vi "Tracker_v2_test_acq_comms_enq.vi"() -> ()   [LabVIEW 2018]
uses:
  Tracker.lvlib
panel:
  out "Data frame":T1
  out "Dequeued data frame":cluster{"String":string, timestamp}
  in  "Play/Pause":bool
  in  "Stop Button":bool
  out "Read buffer":string
  in  "VISA resource name in":refnum<visa-resource-name>="ASRL3::INSTR"
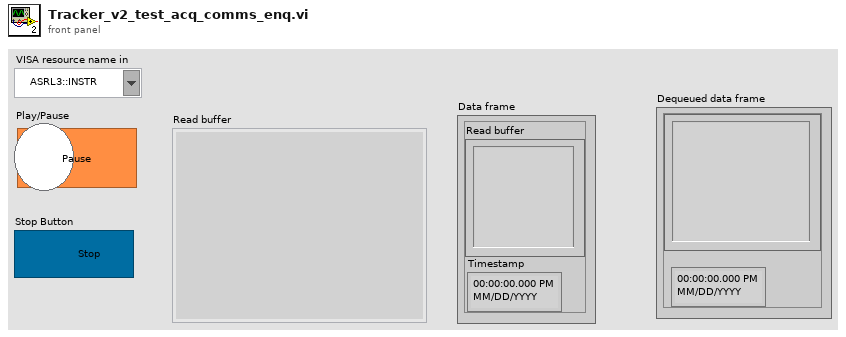
[diagram p1: front panel]
types:
  T1 = cluster{"Read buffer":string, "Timestamp":timestamp}
  T2 = cluster{"Data acquisition status":refnum<notifier>, "Play/Pause status":refnum<notifier>, "Recording status":refnum<notifier>}
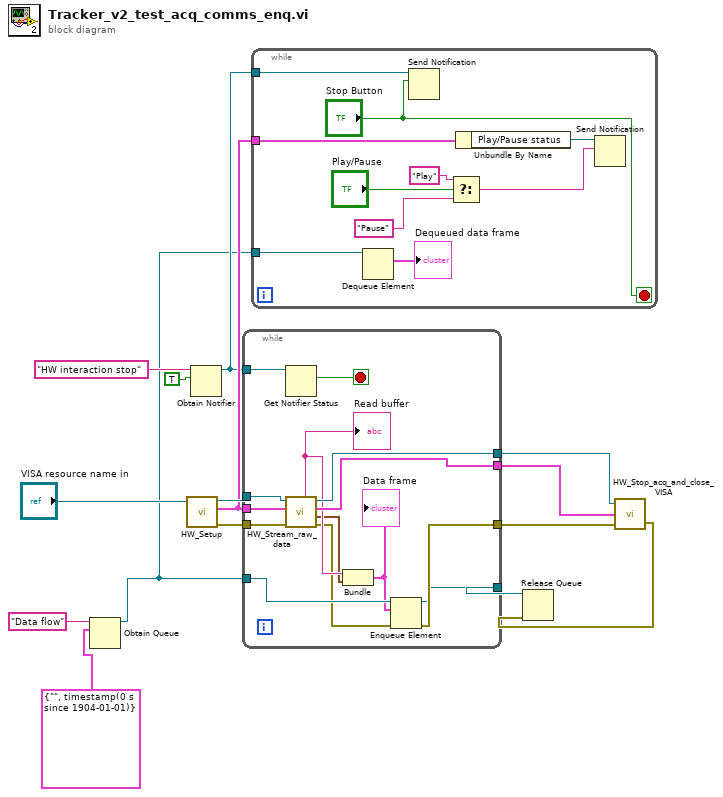
[diagram p0: block diagram]
diagram:
  n1 = Obtain Queue(name (unnamed)="Data flow", element data type=cluster{string, timestamp} {"", timestamp(0 s since 1904-01-01)}) -> (queue out=w6:refnum<queue>)  [unwired: 3 in, 2 out]
  n2 = call "HW_Setup.vi"("VISA resource name in"="VISA resource name in") -> ("VISA resource name out"=w14:refnum<visa-resource-name>, "Data flow controls"=w10:T2, "error out"=w13:errorcluster)  [unwired: 2 in, 1 out]
  n3 = Obtain Notifier(name (unnamed)="HW interaction stop", notification data type=TRUE) -> (notifier out=w7:refnum<notifier>)  [unwired: 2 in, 2 out]
  n4 = while {
    tunnel: w14 -> [w29]
    tunnel: [w26] -> w12
    tunnel: w10 -> [w28]
    tunnel: [w25] -> w11
    tunnel: w13 -> [w27]
    tunnel: [w17] -> w3
    tunnel: w7 -> [w24]
    tunnel: w6 -> [w22]
    tunnel: [w16] -> w4
    stop <- w23 stop-if-true
    n5 = Get Notifier Status(notifier=w24) -> (current notification=w23:bool)  [unwired: 1 in, 4 out]
    n6 = call "HW_Stream_raw_data.vi"("error in"=w27, "Data flow controls"=w28, "VISA resource name in"=w29) -> ("error out"=w18:errorcluster, "Timestamp"=w20:timestamp, "Data flow controls out"=w25:T2, "VISA resource name out"=w26:refnum<visa-resource-name>, "Read buffer"=w21:string)  [unwired: 4 in]
    "Read buffer" <- w21
    n7 = Bundle("Read buffer"=w21, "Timestamp"=w20) -> (w19:T1)  [unwired: 1 in]
    "Data frame" <- w19
    n8 = Enqueue Element(queue=w22, element=w19, error in (no error)=w18) -> (queue out=w16:refnum<queue>, error out=w17:errorcluster)  [unwired: 1 in, 1 out]
  }
  n9 = while {
    tunnel: w10 -> [w39]
    tunnel: w7 -> [w33]
    tunnel: w6 -> [w31]
    stop <- "Stop Button" stop-if-true
    n10 = Dequeue Element(queue=w31) -> (element=→"Dequeued data frame":cluster{string, timestamp})  [unwired: 2 in, 3 out]
    n11 = Send Notification(notification="Stop Button", notifier=w33) -> ()  [unwired: 1 in, 2 out]
    n12 = Select(t="Play", s="Play/Pause", f="Pause") -> (s? t:f=w36:string)
    n13 = Unbundle By Name(w39) -> ("Play/Pause status"=w38:refnum<notifier>)
    n14 = Send Notification(notification=w36, notifier=w38) -> ()  [unwired: 1 in, 2 out]
  }
  n15 = call "HW_Stop_acq_and_close_VISA.vi"("error in"=w3, "Data flow controls in"=w11, "VISA resource name in"=w12) -> ("error out"=w2:errorcluster)  [unwired: 1 out]
  n16 = Release Queue(queue=w4, error in (no error)=w2) -> ()  [unwired: 1 in, 3 out]
